vi "Cuenta total.vi"(8 "error in (no error)":errorcluster, 11 "Mensajes in":refnum<class "Mensajes.lvclass">) -> (0 "error out":errorcluster, 3 "Mensajes out":refnum<class "Mensajes.lvclass">)   [LabVIEW 2020, in "Mensajes.lvlib" / "Mensajes.lvclass"]
uses:
  Mensajes.lvclass
  Mensajes.lvclass/Mensajes.ctl
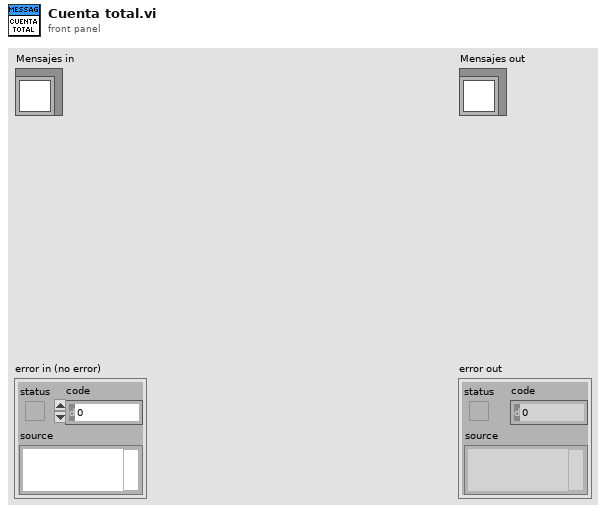
[diagram p1: front panel]
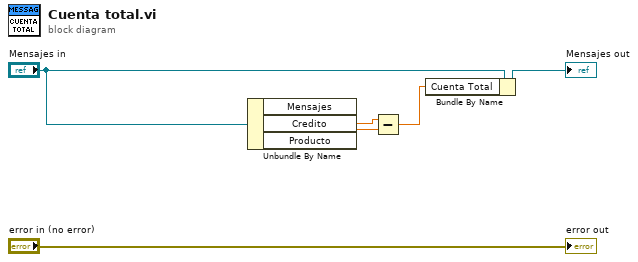
[diagram p0: block diagram]
diagram:
  n1 = Unbundle By Name("Mensajes in") -> ("Credito"=w4:dbl, "Producto"=w3:dbl)  [unwired: 1 out]
  n2 = Subtract(x=w4, y=w3) -> (x-y=w1:dbl)
  n3 = Bundle By Name(cluster="Mensajes in", "Cuenta Total"=w1) -> (→"Mensajes out":refnum<class "Mensajes.lvclass">)
  "error out" <- "error in (no error)"
